vi "EthernetDevice.vi"(0 "Proto":i32(ring) items=["TCP", "UDP", "RTUOverTCP", "RTUOverUDP"], 5 "DeviceID":u8, 7 "Address":string="127.0.0.1", 9 "Port":u16=502) -> (3 "error out":errorcluster, 4 "Device":u64[](array[numeric]))   [LabVIEW 2020, in "SnapMB.lvlib"]
uses:
  SnapMB.lvlib
  windows/snapmb.dll
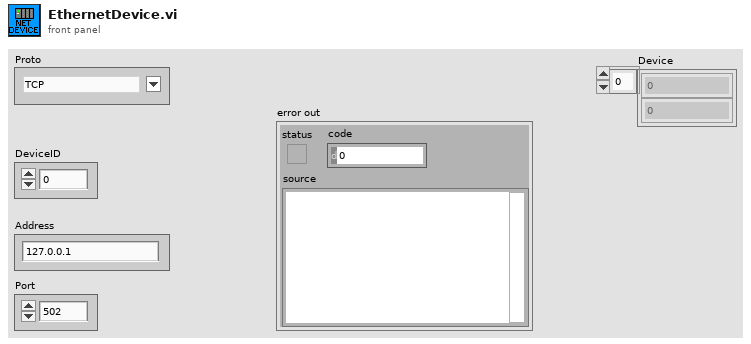
[diagram p1: front panel]
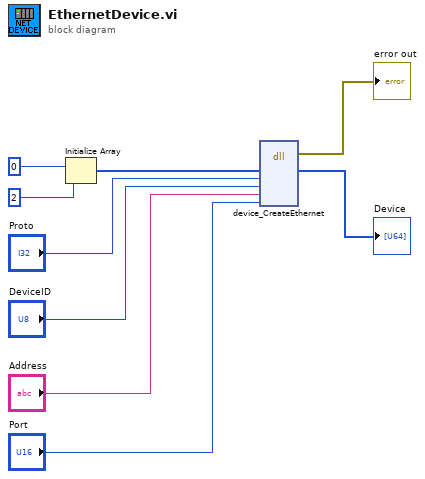
[diagram p0: block diagram]
diagram:
  n1 = Initialize Array(u64 0 ("element"), 2 ("dimension size")) -> (w4:u64[])
  n2 = dll-call lib="D:/SnapMB/LabView/lib/windows/snapmb.dll" fn="device_CreateEthernet"("Device"=w4, "Proto"="Proto", "DeviceID"="DeviceID", "Address"="Address", "Port"="Port") -> (error out=→"error out":errorcluster, "Device"=→"Device":u64[])  [unwired: 8 in, 1 out]
